vi "AlGaInPAs_v19e.vi"(2 "Debug Mode":bool, 3 "Elapsed Time(s)":dbl, 4 "State":enum16{"Edit", "Start", "Run", "End", "Idle"}(ring), 5 "Argument List In":string[](array[string])) -> (0 "Status Out":string, 1 "Argument List Out":string[](array[string]))   [LabVIEW 2011]
uses:
  high_level_proc/Al_bubbler.ctl
  high_level_proc/Ga_bubbler.ctl
  high_level_proc/In_bubbler.ctl
  high_level_proc/P_gas.ctl
  high_level_proc/As_gas.ctl
  high_level_proc/P_bubbler.ctl
panel:
  out "P bubbler Copy":T1 {"P bubbler main"."Flow" format="%.2f"}
  in  "P bubbler":T2 {"P bubbler main"."Flow" format="%.2f"}
  out "As gas Copy":T3 {"As gas main"."Flow" format="%.2f"}
  in  "As gas":T4 {"As gas main"."Flow" format="%.2f"}
  out "P gas Copy":T5 {"P gas main"."Flow" format="%.2f"}
  in  "P gas":T6 {"P gas main"."Flow" format="%.2f"}
  out "In bubbler Copy":T7 {"In main"."Flow" format="%.2f"}
  in  "In bubbler":T8 {"In main"."Flow" format="%.2f"}
  out "Ga bubbler Copy":T9={"Ga bubbler Active"=FALSE, "Ga main"={"Flow"=0.0, "Ga Run"=FALSE, "Prep Ga"=FALSE, "Dilution"=FALSE, "Ga Calculated"=1, "MFC2 flow"=10.0, "MFC3 flow"=100.0, "MFC1 flow"=0.0}} {"Ga main"."MFC1 flow" format="%.4f"; "Ga main"."MFC3 flow" format="%.1f"; "Ga main"."MFC2 flow" format="%.2f"; "Ga main"."Ga Calculated" items=["Ga flow", "MFC1", "MFC2", "MFC3"]; "Ga main"."Flow" format="%.2f"}
  in  "Ga bubbler":T10={"Ga bubbler Active"=FALSE, "Ga main"={"Flow"=0.0, "Ga Run"=FALSE, "Prep Ga"=FALSE, "Dilution"=FALSE, "Ga Calculated"=1, "MFC2 flow"=10.0, "MFC3 flow"=100.0, "MFC1 flow"=0.0}} {"Ga main"."MFC1 flow" format="%.4f"; "Ga main"."MFC3 flow" format="%.1f"; "Ga main"."MFC2 flow" format="%.2f"; "Ga main"."Ga Calculated" items=["Ga flow", "MFC1", "MFC2", "MFC3"]; "Ga main"."Flow" format="%.2f"}
  out "Al bubbler Copy":T11 {"Al main"."Al Flow" format="%.2f"}
  in  "Al bubbler":T12 {"Al main"."Al Flow" format="%.2f"}
  out "prep_done":bool
  out "run started":bool
  out "first":bool=TRUE
  out "total time":dbl
  out "is OK?":bool
  in  "prep_time":dbl
  in  "Cancel":bool
  in  "OK":bool
  out "tTotal(s) 2":dbl
  # "Add pre-run time to run time in editor."
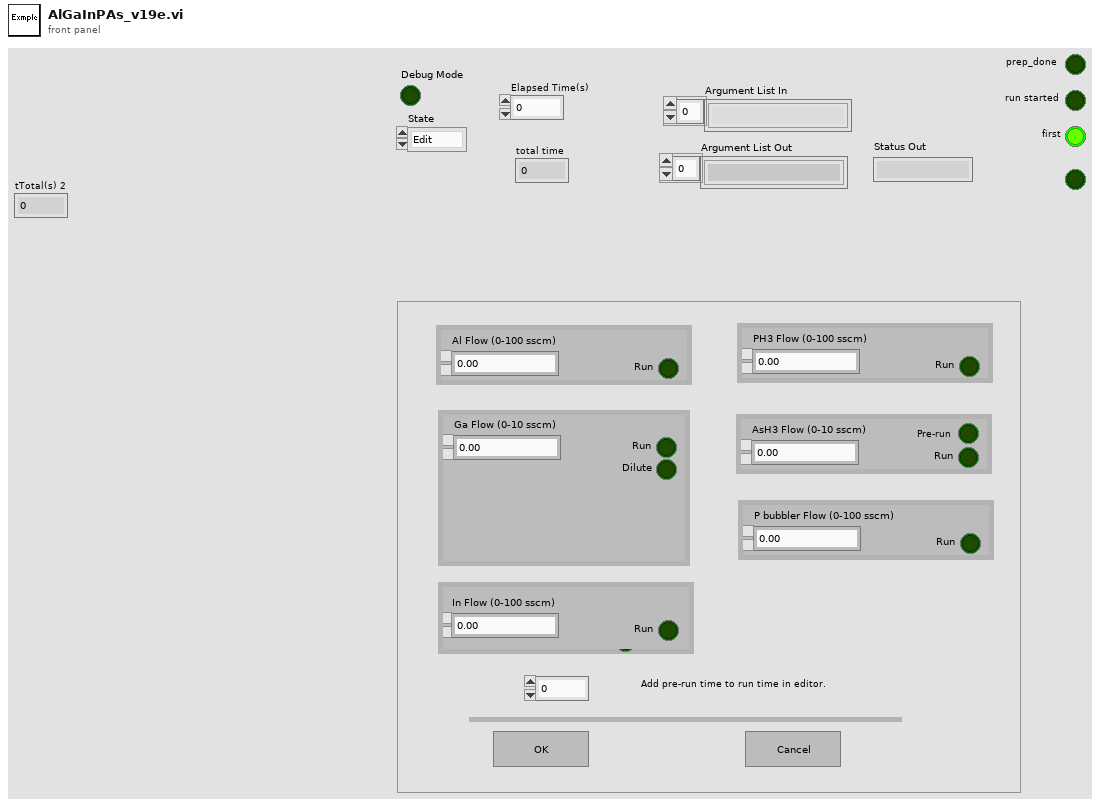
[diagram p1: front panel]
types:
  T1 = cluster{"P bubbler Active":bool, "P bubbler main":cluster{"Flow":dbl, "P bubbler Run":bool, "P bubbler Prep":bool}}
  T2 = typedef "P_bubbler.ctl" = cluster{"P bubbler Active":bool, "P bubbler main":cluster{"Flow":dbl, "P bubbler Run":bool, "P bubbler Prep":bool}}
  T3 = cluster{"As gas Active":bool, "As gas main":cluster{"Flow":dbl, "AsH3 Run":bool, "AsH3 Prep":bool}}
  T4 = typedef "As_gas.ctl" = cluster{"As gas Active":bool, "As gas main":cluster{"Flow":dbl, "AsH3 Run":bool, "AsH3 Prep":bool}}
  T5 = cluster{"P gas Active":bool, "P gas main":cluster{"Flow":dbl, "PH3 Run":bool, "PH3 Prep":bool}}
  T6 = typedef "P_gas.ctl" = cluster{"P gas Active":bool, "P gas main":cluster{"Flow":dbl, "PH3 Run":bool, "PH3 Prep":bool}}
  T7 = cluster{"In main":cluster{"Flow":dbl, "In Run":bool, "Prep In":bool}, "In bubbler Active":bool}
  T8 = typedef "In_bubbler.ctl" = cluster{"In main":cluster{"Flow":dbl, "In Run":bool, "Prep In":bool}, "In bubbler Active":bool}
  T9 = cluster{"Ga bubbler Active":bool, "Ga main":cluster{"Flow":dbl, "Ga Run":bool, "Prep Ga":bool, "Dilution":bool, "Ga Calculated":u16, "MFC2 flow":dbl, "MFC3 flow":dbl, "MFC1 flow":dbl}}
  T10 = typedef "Ga_bubbler.ctl" = cluster{"Ga bubbler Active":bool, "Ga main":cluster{"Flow":dbl, "Ga Run":bool, "Prep Ga":bool, "Dilution":bool, "Ga Calculated":u16, "MFC2 flow":dbl, "MFC3 flow":dbl, "MFC1 flow":dbl}}
  T11 = cluster{"Al Active":bool, "Al main":cluster{"Al Flow":dbl, "Al Run":bool, "Prep Al":bool}}
  T12 = typedef "Al_bubbler.ctl" = cluster{"Al Active":bool, "Al main":cluster{"Al Flow":dbl, "Al Run":bool, "Prep Al":bool}}
  T13 = enum16{"Discrete", "Continuous", "Instantaneous", "Finite"}
  T14 = enum32{"Invalid", "Default", "Floating", "Floating/Auto-Hide", "Modal"}
  T15 = enum8{"Enabled", "Disabled", "Disabled and Grayed Out"}
  T16 = cluster{"Al Flow":dbl, "Al Run":bool, "Prep Al":bool}
  T17 = cluster{"Flow":dbl, "Ga Run":bool, "Prep Ga":bool, "Dilution":bool, "Ga Calculated":u16, "MFC2 flow":dbl, "MFC3 flow":dbl, "MFC1 flow":dbl}
  T18 = cluster{"Flow":dbl, "In Run":bool, "Prep In":bool}
  T19 = cluster{"Flow":dbl, "PH3 Run":bool, "PH3 Prep":bool}
  T20 = cluster{"Flow":dbl, "AsH3 Run":bool, "AsH3 Prep":bool}
  T21 = cluster{"Flow":dbl, "P bubbler Run":bool, "P bubbler Prep":bool}
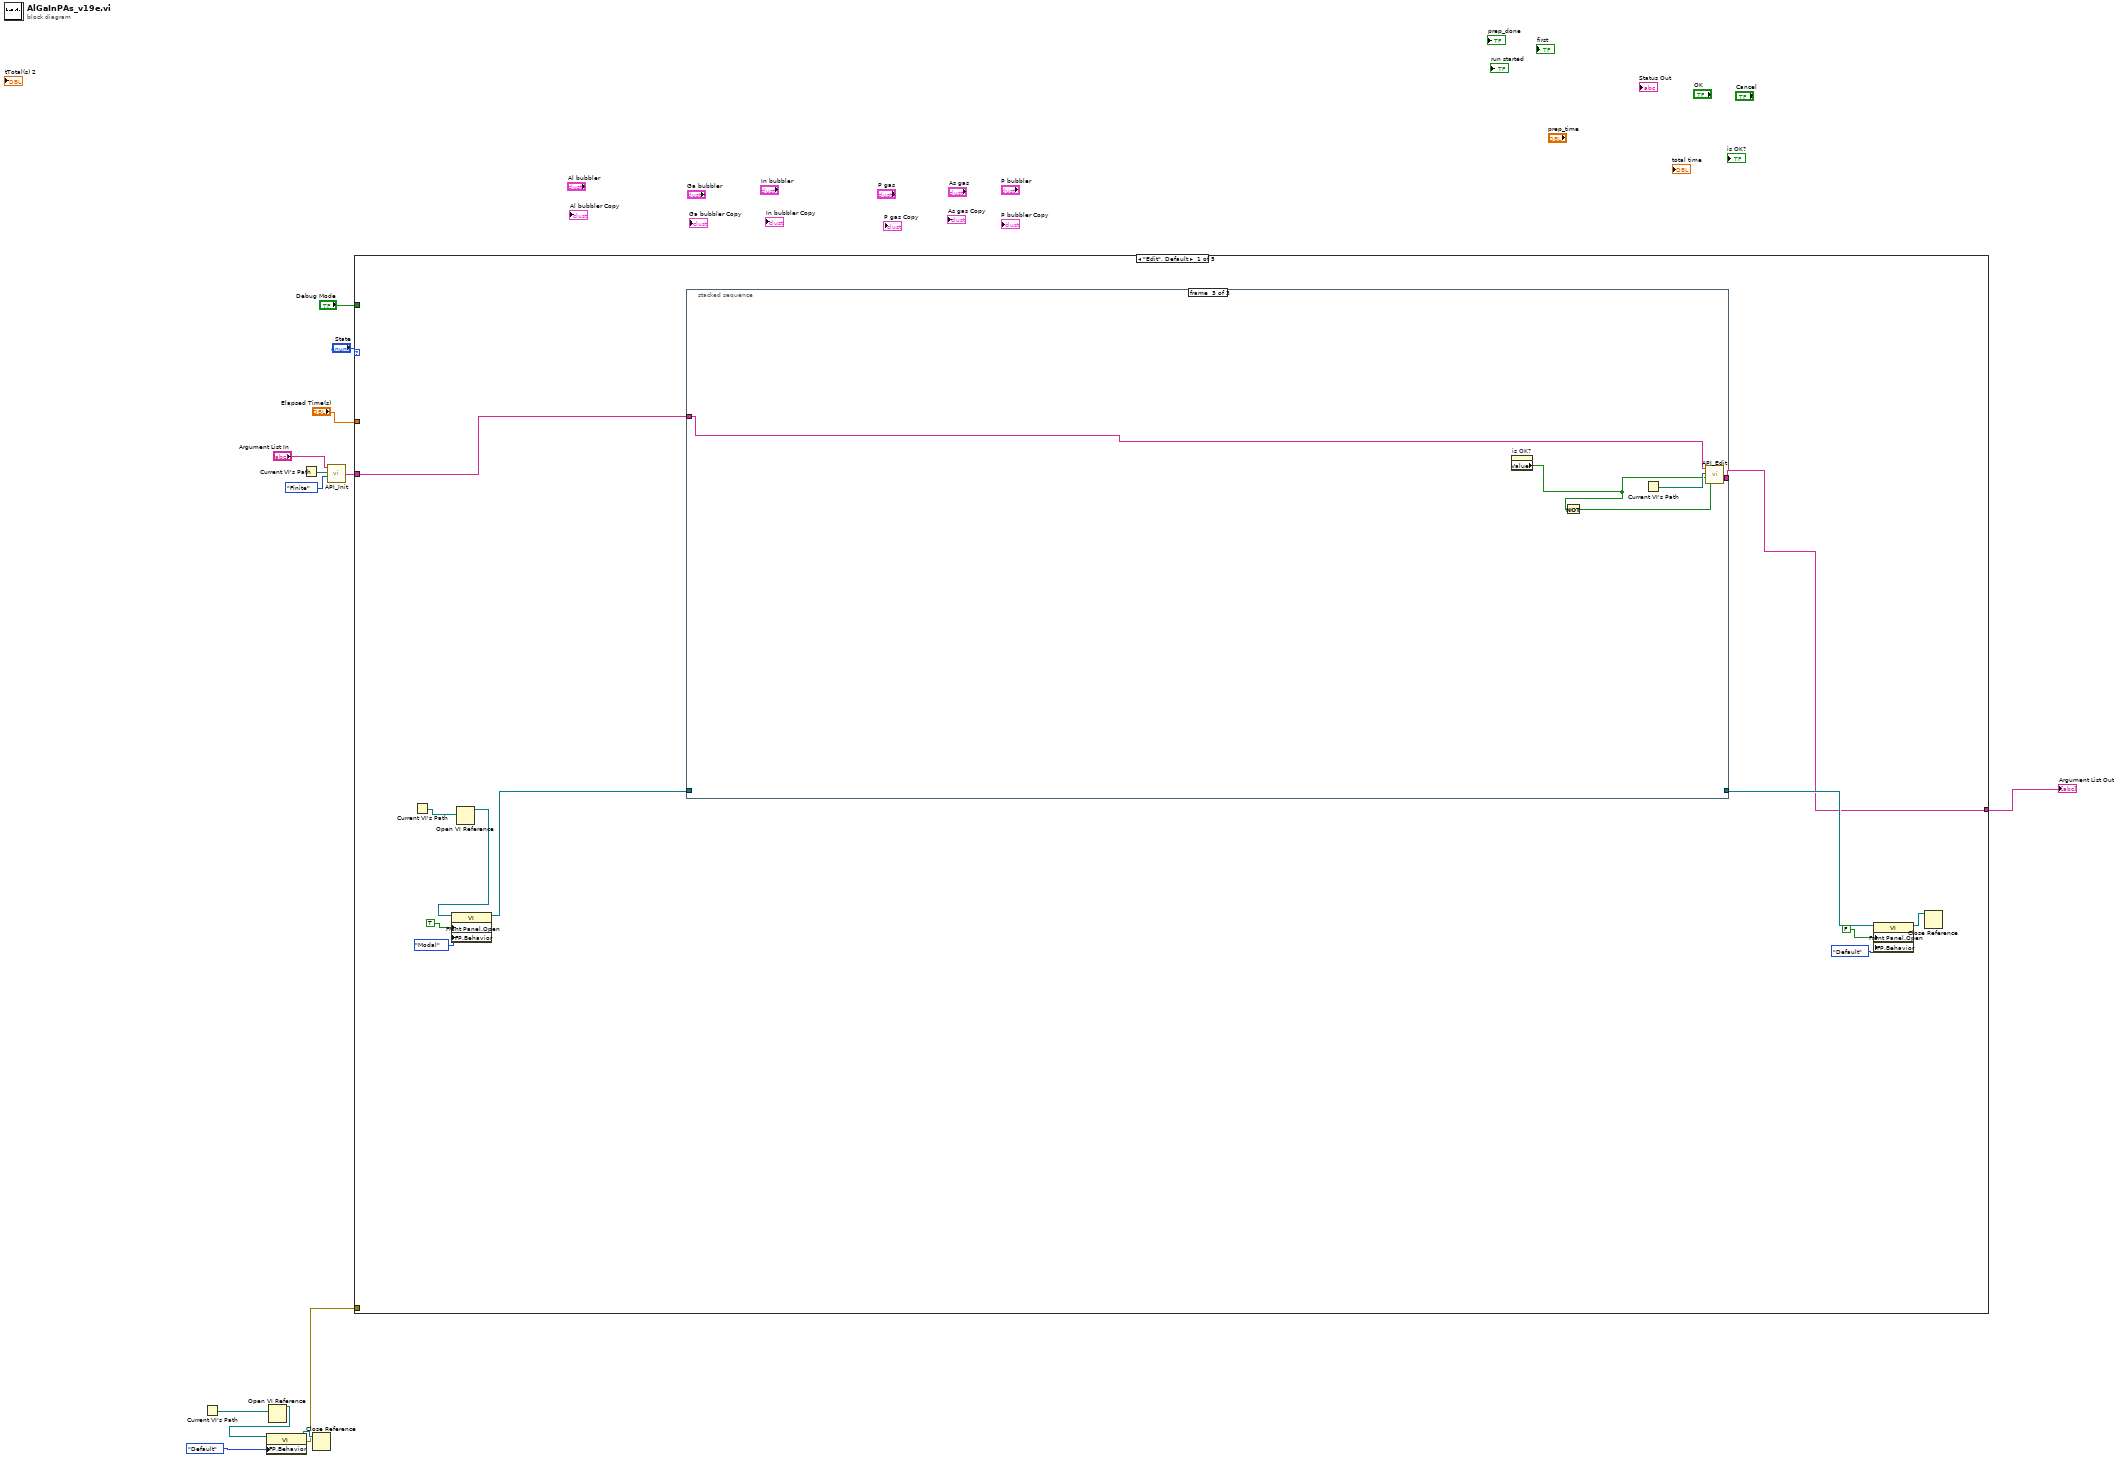
[diagram p0: block diagram]
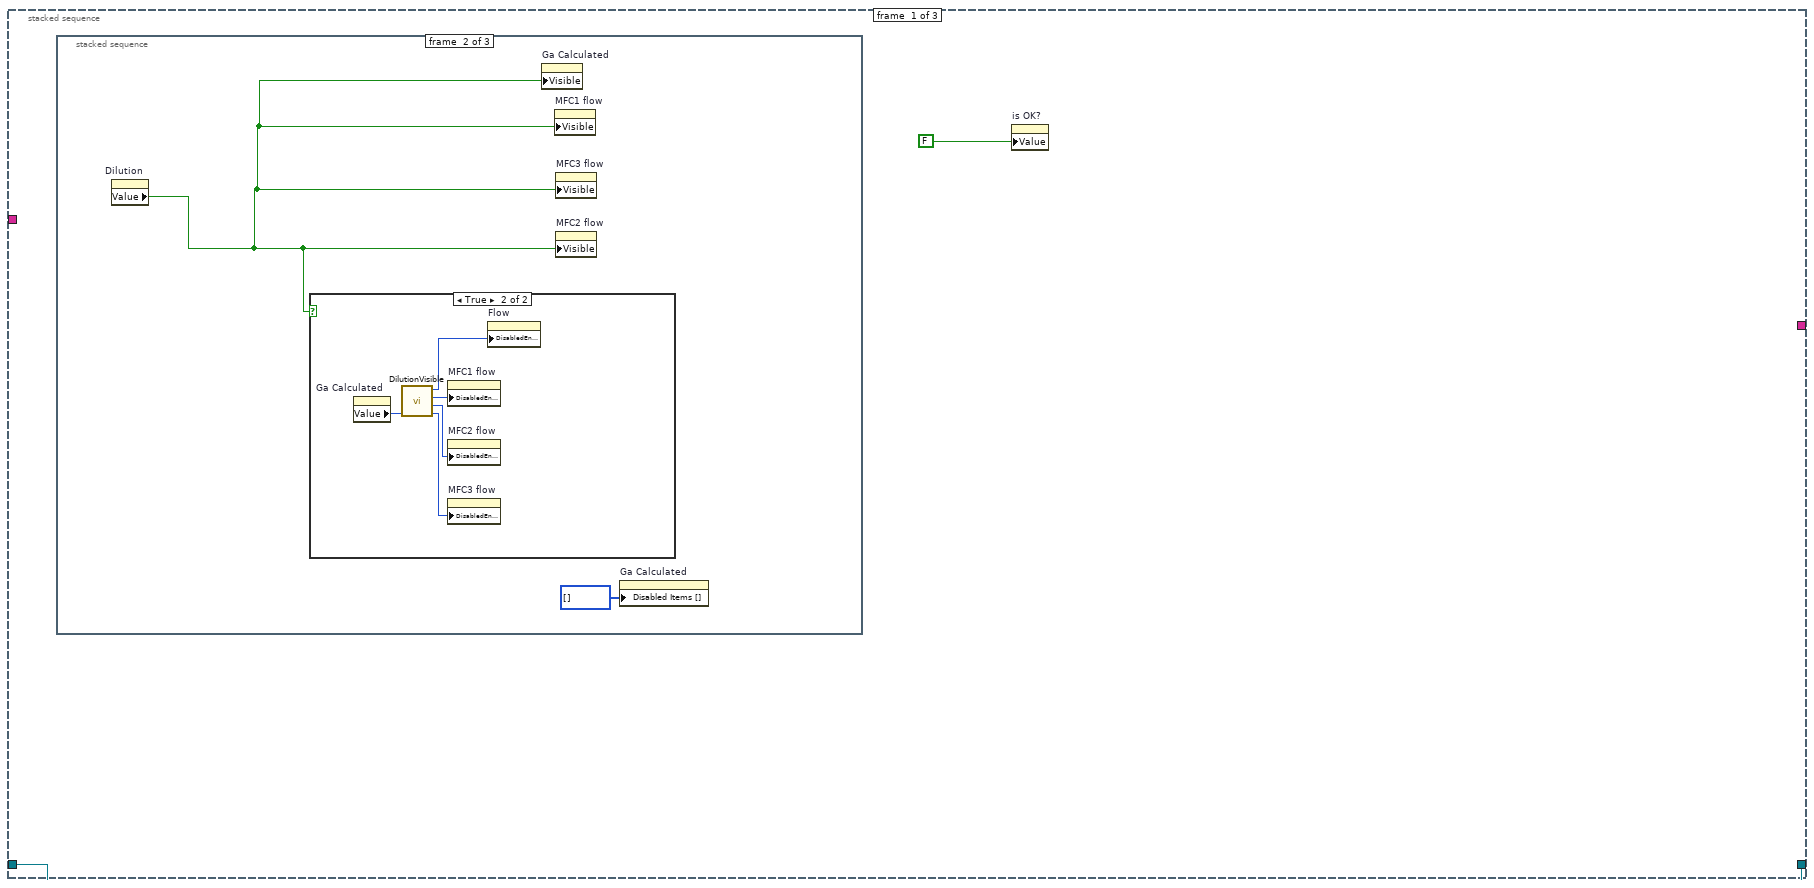
[diagram p2: hidden frame]
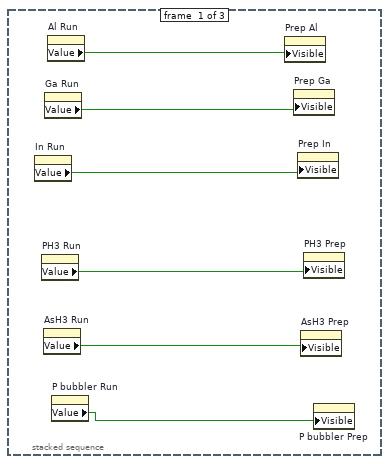
[diagram p3: hidden frame]
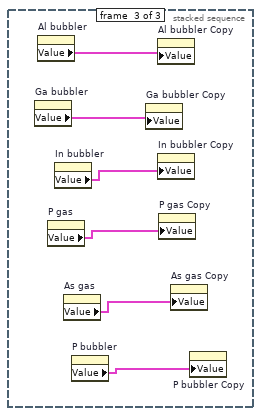
[diagram p5: hidden frame]
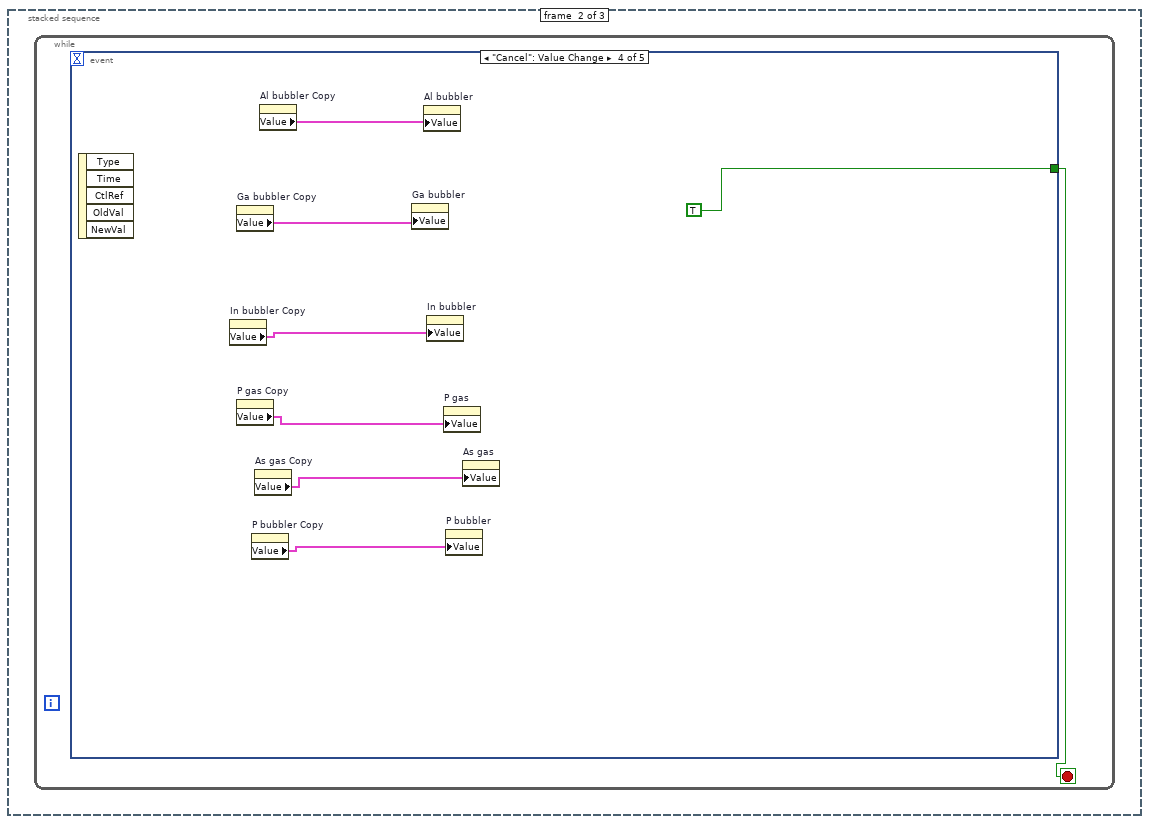
[diagram p6: hidden frame]
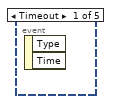
[diagram p7: hidden frame]
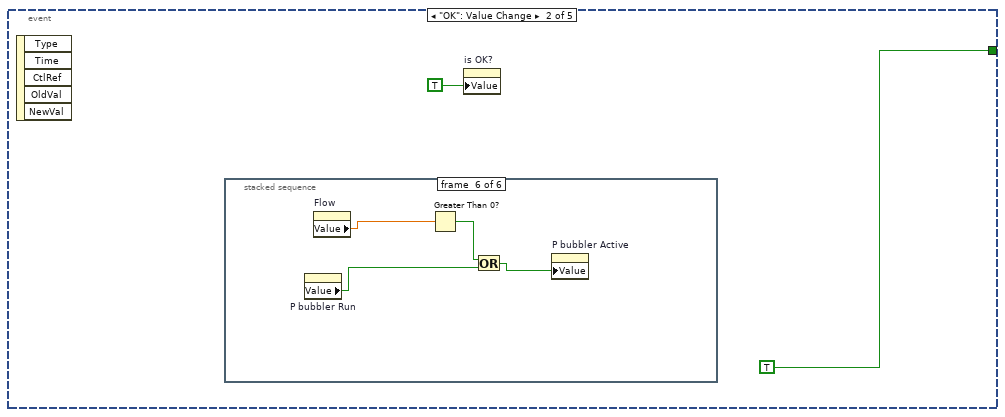
[diagram p8: hidden frame]
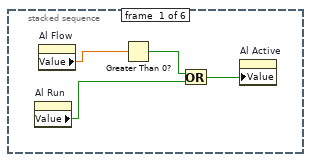
[diagram p9: hidden frame]
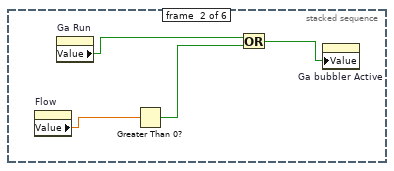
[diagram p10: hidden frame]
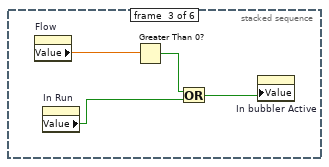
[diagram p11: hidden frame]
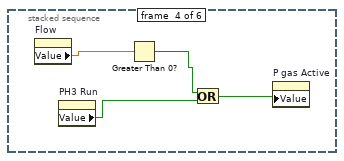
[diagram p12: hidden frame]
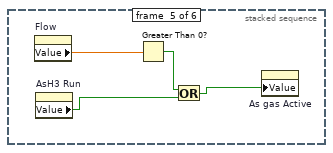
[diagram p13: hidden frame]
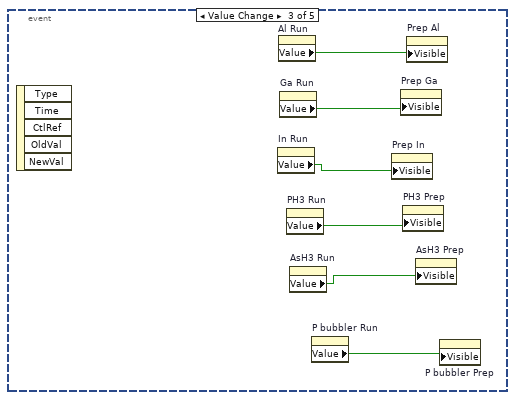
[diagram p14: hidden frame]
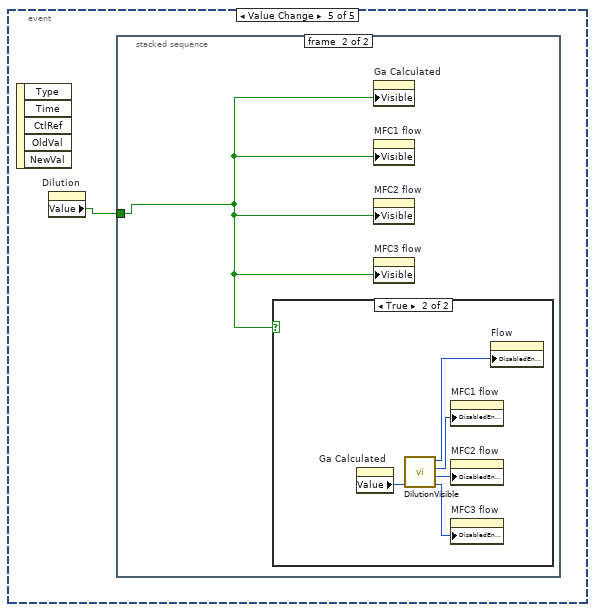
[diagram p15: hidden frame]
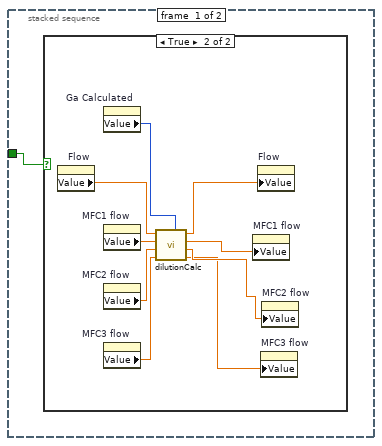
[diagram p16: hidden frame]
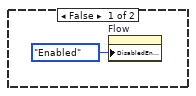
[diagram p18: hidden frame]
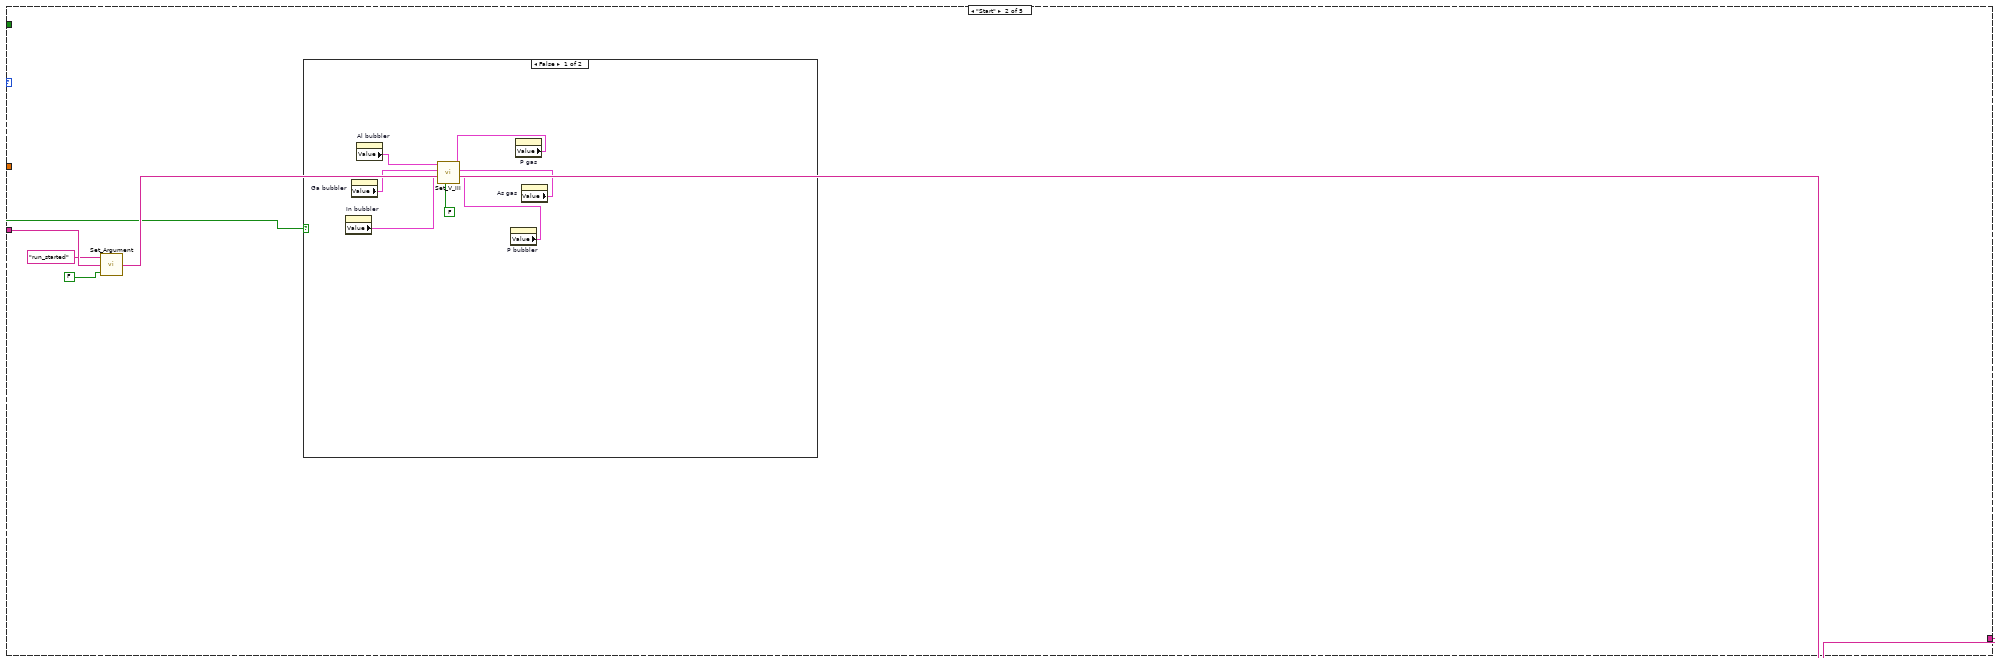
[diagram p19: hidden frame]
diagram:
  n1 = Current VI's Path() -> (path=w9:path)
  n2 = Open VI Reference(vi path=w9) -> (vi reference=w8:refnum<vi>)  [unwired: 1 in, 5 out]
  n3 = property class="VI"(reference=w8, "FP.Behavior"=T14."Default" ("Front Panel Window:Behavior")) -> (reference out=w6:refnum<vi>, error out=w5:errorcluster)  [unwired: 1 in]
  n4 = Current VI's Path() -> (path=w4:path)
  n5 = Close Reference(reference=w6) -> ()  [unwired: 1 in, 1 out]
  n6 = call "API_Init.vi"("API Mode"=T13."Finite", "VI Path"=w4, "Argument List In"="Argument List In") -> ("Argument List Out"=w1:string[])  [unwired: 1 in]
  n7 = case shown="\"Edit\", Default" "State" {
    tunnel: "Debug Mode" -> [_ w109 w123 _ _]
    tunnel: "Elapsed Time(s)" -> [_ _ w124 _ _]
    tunnel: w1 -> [w15 w111 w122 w222 w223]
    tunnel: [w14 w110 w121 w222 w223] -> w10
    tunnel: w5 -> [_ _ _ _ _]
    frame "Edit", Default {
      n8 = Current VI's Path() -> (path=w20:path)
      n9 = Open VI Reference(vi path=w20) -> (vi reference=w19:refnum<vi>)  [unwired: 1 in, 5 out]
      n10 = property class="VI"(reference=w19, "Front Panel.Open"=TRUE ("Front Panel Window:Open"), "FP.Behavior"=T14."Modal" ("Front Panel Window:Behavior")) -> (reference out=w18:refnum<vi>)  [unwired: 1 in, 1 out]
      n11 = stacked-sequence {
        tunnel: w15 -> [_ _ w105]
        tunnel: w18 -> [w26 _ _]
        tunnel: [w26 _ _] -> w22
        tunnel: [_ _ w106] -> w14
        frame #0 {
          n12 = stacked-sequence {
            frame #0 {
              n13 = property on="In Run" class="Bool (strict)"() -> ("Value"=w31:bool)  [unwired: 2 in, 2 out]
              n14 = property on="PH3 Run" class="Bool (strict)"() -> ("Value"=w29:bool)  [unwired: 2 in, 2 out]
              n15 = property on="AsH3 Run" class="Bool (strict)"() -> ("Value"=w28:bool)  [unwired: 2 in, 2 out]
              n16 = property on="Ga Run" class="Bool (strict)"() -> ("Value"=w30:bool)  [unwired: 2 in, 2 out]
              n17 = property on="Al Run" class="Bool (strict)"() -> ("Value"=w32:bool)  [unwired: 2 in, 2 out]
              n18 = property on="P bubbler Run" class="Bool (strict)"() -> ("Value"=w27:bool)  [unwired: 2 in, 2 out]
              n19 = property on="Prep Al" class="Bool (strict)"("Visible"=w32) -> ()  [unwired: 2 in, 2 out]
              n20 = property on="Prep Ga" class="Bool (strict)"("Visible"=w30) -> ()  [unwired: 2 in, 2 out]
              n21 = property on="Prep In" class="Bool (strict)"("Visible"=w31) -> ()  [unwired: 2 in, 2 out]
              n22 = property on="AsH3 Prep" class="Bool (strict)"("Visible"=w28) -> ()  [unwired: 2 in, 2 out]
              n23 = property on="PH3 Prep" class="Bool (strict)"("Visible"=w29) -> ()  [unwired: 2 in, 2 out]
              n24 = property on="P bubbler Prep" class="Bool (strict)"("Visible"=w27) -> ()  [unwired: 2 in, 2 out]
            }
            frame #1 {
              n25 = property on="Dilution" class="Bool (strict)"() -> ("Value"=w34:bool)  [unwired: 2 in, 2 out]
              n26 = case shown="True" w34 {
                frame False {
                }
                frame True {
                  n27 = property on="Ga Calculated" class="Ring (strict)"() -> ("Value"=w35:u16)  [unwired: 2 in, 2 out]
                  n28 = call "DilutionVisible.vi"("calculated"=w35) -> ("MFC3"=w38:u16, "MFC2"=w37:u16, "MFC1"=w36:u16, "flow"=w39:u16)  [unwired: 3 in]
                  n29 = property on="MFC1 flow" class="DigNum (strict)"("DisabledEnum"=w36) -> ()  [unwired: 2 in, 2 out]
                  n30 = property on="MFC2 flow" class="DigNum (strict)"("DisabledEnum"=w37) -> ()  [unwired: 2 in, 2 out]
                  n31 = property on="MFC3 flow" class="DigNum (strict)"("DisabledEnum"=w38) -> ()  [unwired: 2 in, 2 out]
                  n32 = property on="Flow" class="DigNum (strict)"("DisabledEnum"=w39) -> ()  [unwired: 2 in, 2 out]
                }
              }
              n33 = property on="Ga Calculated" class="Ring (strict)"("Visible"=w34) -> ()  [unwired: 2 in, 2 out]
              n34 = property on="MFC1 flow" class="DigNum (strict)"("Visible"=w34) -> ()  [unwired: 2 in, 2 out]
              n35 = property on="MFC3 flow" class="DigNum (strict)"("Visible"=w34) -> ()  [unwired: 2 in, 2 out]
              n36 = property on="MFC2 flow" class="DigNum (strict)"("Visible"=w34) -> ()  [unwired: 2 in, 2 out]
              n37 = property on="Ga Calculated" class="Ring (strict)"("Disabled Items []"=i32[] []) -> ()  [unwired: 2 in, 2 out]
            }
            frame #2 {
              n38 = property on="Ga bubbler" class="Clust (strict)"() -> ("Value"=w44:T9)  [unwired: 2 in, 2 out]
              n39 = property on="Al bubbler" class="Clust (strict)"() -> ("Value"=w45:T11)  [unwired: 2 in, 2 out]
              n40 = property on="P gas" class="Clust (strict)"() -> ("Value"=w42:T5)  [unwired: 2 in, 2 out]
              n41 = property on="In bubbler" class="Clust (strict)"() -> ("Value"=w43:T7)  [unwired: 2 in, 2 out]
              n42 = property on="As gas" class="Clust (strict)"() -> ("Value"=w41:T3)  [unwired: 2 in, 2 out]
              n43 = property on="P bubbler" class="Clust (strict)"() -> ("Value"=w40:T1)  [unwired: 2 in, 2 out]
              n44 = property on="Ga bubbler Copy" class="Clust (strict)"("Value"=w44) -> ()  [unwired: 2 in, 2 out]
              n45 = property on="Al bubbler Copy" class="Clust (strict)"("Value"=w45) -> ()  [unwired: 2 in, 2 out]
              n46 = property on="In bubbler Copy" class="Clust (strict)"("Value"=w43) -> ()  [unwired: 2 in, 2 out]
              n47 = property on="P gas Copy" class="Clust (strict)"("Value"=w42) -> ()  [unwired: 2 in, 2 out]
              n48 = property on="As gas Copy" class="Clust (strict)"("Value"=w41) -> ()  [unwired: 2 in, 2 out]
              n49 = property on="P bubbler Copy" class="Clust (strict)"("Value"=w40) -> ()  [unwired: 2 in, 2 out]
            }
          }
          n50 = property on="is OK?" class="Bool (strict)"("Value"=FALSE ("is OK?")) -> ()  [unwired: 2 in, 2 out]
        }
        frame #1 {
          n51 = while {
            stop <- w46 stop-if-true
            n52 = event shown="[3] \"Cancel\": Value Change" {
              selector: _ -> [_ _ _ _ _]
              dyn-events: _ -> [_ _ _ _ _]
              timeout: _ -> [_ _ _ _ _]
              tunnel: [_ TRUE _ TRUE _] -> w46
              event Timeout {
                n53 = event-data() -> ()  [unwired: 1 in, 2 out]
              }
              event "OK": Value Change {
                n54 = event-data() -> ()  [unwired: 1 in, 5 out]
                n55 = stacked-sequence {
                  frame #0 {
                    n56 = property on="Al Run" class="Bool (strict)"() -> ("Value"=w50:bool)  [unwired: 2 in, 2 out]
                    n57 = property on="Al Flow" class="DigNum (strict)"() -> ("Value"=w51:dbl)  [unwired: 2 in, 2 out]
                    n58 = Greater Than 0?(x=w51) -> (x > 0?=w52:bool)
                    n59 = Or(x=w52, y=w50) -> (x .or. y?=w49:bool)
                    n60 = property on="Al Active" class="Bool (strict)"("Value"=w49) -> ()  [unwired: 2 in, 2 out]
                  }
                  frame #1 {
                    n61 = property on="Flow" class="DigNum (strict)"() -> ("Value"=w53:dbl)  [unwired: 2 in, 2 out]
                    n62 = property on="Ga Run" class="Bool (strict)"() -> ("Value"=w54:bool)  [unwired: 2 in, 2 out]
                    n63 = Greater Than 0?(x=w53) -> (x > 0?=w56:bool)
                    n64 = Or(x=w54, y=w56) -> (x .or. y?=w55:bool)
                    n65 = property on="Ga bubbler Active" class="Bool (strict)"("Value"=w55) -> ()  [unwired: 2 in, 2 out]
                  }
                  frame #2 {
                    n66 = property on="Flow" class="DigNum (strict)"() -> ("Value"=w59:dbl)  [unwired: 2 in, 2 out]
                    n67 = property on="In Run" class="Bool (strict)"() -> ("Value"=w58:bool)  [unwired: 2 in, 2 out]
                    n68 = Greater Than 0?(x=w59) -> (x > 0?=w60:bool)
                    n69 = Or(x=w60, y=w58) -> (x .or. y?=w57:bool)
                    n70 = property on="In bubbler Active" class="Bool (strict)"("Value"=w57) -> ()  [unwired: 2 in, 2 out]
                  }
                  frame #3 {
                    n71 = property on="Flow" class="DigNum (strict)"() -> ("Value"=w63:dbl)  [unwired: 2 in, 2 out]
                    n72 = property on="PH3 Run" class="Bool (strict)"() -> ("Value"=w62:bool)  [unwired: 2 in, 2 out]
                    n73 = Greater Than 0?(x=w63) -> (x > 0?=w64:bool)
                    n74 = Or(x=w64, y=w62) -> (x .or. y?=w61:bool)
                    n75 = property on="P gas Active" class="Bool (strict)"("Value"=w61) -> ()  [unwired: 2 in, 2 out]
                  }
                  frame #4 {
                    n76 = property on="Flow" class="DigNum (strict)"() -> ("Value"=w67:dbl)  [unwired: 2 in, 2 out]
                    n77 = property on="AsH3 Run" class="Bool (strict)"() -> ("Value"=w66:bool)  [unwired: 2 in, 2 out]
                    n78 = Greater Than 0?(x=w67) -> (x > 0?=w68:bool)
                    n79 = Or(x=w68, y=w66) -> (x .or. y?=w65:bool)
                    n80 = property on="As gas Active" class="Bool (strict)"("Value"=w65) -> ()  [unwired: 2 in, 2 out]
                  }
                  frame #5 {
                    n81 = property on="P bubbler Run" class="Bool (strict)"() -> ("Value"=w70:bool)  [unwired: 2 in, 2 out]
                    n82 = property on="Flow" class="DigNum (strict)"() -> ("Value"=w71:dbl)  [unwired: 2 in, 2 out]
                    n83 = Greater Than 0?(x=w71) -> (x > 0?=w72:bool)
                    n84 = Or(x=w72, y=w70) -> (x .or. y?=w69:bool)
                    n85 = property on="P bubbler Active" class="Bool (strict)"("Value"=w69) -> ()  [unwired: 2 in, 2 out]
                  }
                }
                n86 = property on="is OK?" class="Bool (strict)"("Value"=TRUE ("is OK?")) -> ()  [unwired: 2 in, 2 out]
              }
              event Value Change {
                n87 = event-data() -> ()  [unwired: 1 in, 5 out]
                n88 = property on="In Run" class="Bool (strict)"() -> ("Value"=w75:bool)  [unwired: 2 in, 2 out]
                n89 = property on="Al Run" class="Bool (strict)"() -> ("Value"=w77:bool)  [unwired: 2 in, 2 out]
                n90 = property on="Ga Run" class="Bool (strict)"() -> ("Value"=w76:bool)  [unwired: 2 in, 2 out]
                n91 = property on="PH3 Run" class="Bool (strict)"() -> ("Value"=w74:bool)  [unwired: 2 in, 2 out]
                n92 = property on="AsH3 Run" class="Bool (strict)"() -> ("Value"=w73:bool)  [unwired: 2 in, 2 out]
                n93 = property on="P bubbler Run" class="Bool (strict)"() -> ("Value"=w78:bool)  [unwired: 2 in, 2 out]
                n94 = property on="Prep In" class="Bool (strict)"("Visible"=w75) -> ()  [unwired: 2 in, 2 out]
                n95 = property on="Prep Ga" class="Bool (strict)"("Visible"=w76) -> ()  [unwired: 2 in, 2 out]
                n96 = property on="PH3 Prep" class="Bool (strict)"("Visible"=w74) -> ()  [unwired: 2 in, 2 out]
                n97 = property on="Prep Al" class="Bool (strict)"("Visible"=w77) -> ()  [unwired: 2 in, 2 out]
                n98 = property on="AsH3 Prep" class="Bool (strict)"("Visible"=w73) -> ()  [unwired: 2 in, 2 out]
                n99 = property on="P bubbler Prep" class="Bool (strict)"("Visible"=w78) -> ()  [unwired: 2 in, 2 out]
              }
              event "Cancel": Value Change {
                n100 = event-data() -> ()  [unwired: 1 in, 5 out]
                n101 = property on="In bubbler Copy" class="Clust (strict)"() -> ("Value"=w83:T7)  [unwired: 2 in, 2 out]
                n102 = property on="Ga bubbler Copy" class="Clust (strict)"() -> ("Value"=w82:T9)  [unwired: 2 in, 2 out]
                n103 = property on="P gas Copy" class="Clust (strict)"() -> ("Value"=w81:T5)  [unwired: 2 in, 2 out]
                n104 = property on="P bubbler Copy" class="Clust (strict)"() -> ("Value"=w79:T1)  [unwired: 2 in, 2 out]
                n105 = property on="As gas Copy" class="Clust (strict)"() -> ("Value"=w80:T3)  [unwired: 2 in, 2 out]
                n106 = property on="Al bubbler Copy" class="Clust (strict)"() -> ("Value"=w84:T11)  [unwired: 2 in, 2 out]
                n107 = property on="Ga bubbler" class="Clust (strict)"("Value"=w82) -> ()  [unwired: 2 in, 2 out]
                n108 = property on="Al bubbler" class="Clust (strict)"("Value"=w84) -> ()  [unwired: 2 in, 2 out]
                n109 = property on="In bubbler" class="Clust (strict)"("Value"=w83) -> ()  [unwired: 2 in, 2 out]
                n110 = property on="P gas" class="Clust (strict)"("Value"=w81) -> ()  [unwired: 2 in, 2 out]
                n111 = property on="P bubbler" class="Clust (strict)"("Value"=w79) -> ()  [unwired: 2 in, 2 out]
                n112 = property on="As gas" class="Clust (strict)"("Value"=w80) -> ()  [unwired: 2 in, 2 out]
              }
              event Value Change {
                n113 = event-data() -> ()  [unwired: 1 in, 5 out]
                n114 = property on="Dilution" class="Bool (strict)"() -> ("Value"=w86:bool)  [unwired: 2 in, 2 out]
                n115 = stacked-sequence {
                  tunnel: w86 -> [w87 w97]
                  frame #0 {
                    n116 = case shown="True" w87 {
                      frame False {
                      }
                      frame True {
                        n117 = property on="Flow" class="DigNum (strict)"() -> ("Value"=w95:dbl)  [unwired: 2 in, 2 out]
                        n118 = property on="Ga Calculated" class="Ring (strict)"() -> ("Value"=w96:u16)  [unwired: 2 in, 2 out]
                        n119 = property on="MFC1 flow" class="DigNum (strict)"() -> ("Value"=w94:dbl)  [unwired: 2 in, 2 out]
                        n120 = property on="MFC2 flow" class="DigNum (strict)"() -> ("Value"=w93:dbl)  [unwired: 2 in, 2 out]
                        n121 = property on="MFC3 flow" class="DigNum (strict)"() -> ("Value"=w92:dbl)  [unwired: 2 in, 2 out]
                        n122 = call "dilutionCalc.vi"("Calculated"=w96, "MFC3"=w92, "MFC2"=w93, "MFC1"=w94, "flow"=w95) -> ("MFC3 out"=w88:dbl, "MFC2 out"=w89:dbl, "MFC1 out"=w90:dbl, "flow out"=w91:dbl)  [unwired: 1 in]
                        n123 = property on="MFC1 flow" class="DigNum (strict)"("Value"=w90) -> ()  [unwired: 2 in, 2 out]
                        n124 = property on="Flow" class="DigNum (strict)"("Value"=w91) -> ()  [unwired: 2 in, 2 out]
                        n125 = property on="MFC3 flow" class="DigNum (strict)"("Value"=w88) -> ()  [unwired: 2 in, 2 out]
                        n126 = property on="MFC2 flow" class="DigNum (strict)"("Value"=w89) -> ()  [unwired: 2 in, 2 out]
                      }
                    }
                  }
                  frame #1 {
                    n127 = case shown="True" w97 {
                      frame False {
                        n128 = property on="Flow" class="DigNum (strict)"("DisabledEnum"=T15."Enabled" ("Disabled")) -> ()  [unwired: 2 in, 2 out]
                      }
                      frame True {
                        n129 = property on="Ga Calculated" class="Ring (strict)"() -> ("Value"=w99:u16)  [unwired: 2 in, 2 out]
                        n130 = call "DilutionVisible.vi"("calculated"=w99) -> ("MFC3"=w103:u16, "MFC2"=w102:u16, "MFC1"=w101:u16, "flow"=w100:u16)  [unwired: 3 in]
                        n131 = property on="MFC1 flow" class="DigNum (strict)"("DisabledEnum"=w101) -> ()  [unwired: 2 in, 2 out]
                        n132 = property on="MFC2 flow" class="DigNum (strict)"("DisabledEnum"=w102) -> ()  [unwired: 2 in, 2 out]
                        n133 = property on="MFC3 flow" class="DigNum (strict)"("DisabledEnum"=w103) -> ()  [unwired: 2 in, 2 out]
                        n134 = property on="Flow" class="DigNum (strict)"("DisabledEnum"=w100) -> ()  [unwired: 2 in, 2 out]
                      }
                    }
                    n135 = property on="Ga Calculated" class="Ring (strict)"("Visible"=w97) -> ()  [unwired: 2 in, 2 out]
                    n136 = property on="MFC1 flow" class="DigNum (strict)"("Visible"=w97) -> ()  [unwired: 2 in, 2 out]
                    n137 = property on="MFC2 flow" class="DigNum (strict)"("Visible"=w97) -> ()  [unwired: 2 in, 2 out]
                    n138 = property on="MFC3 flow" class="DigNum (strict)"("Visible"=w97) -> ()  [unwired: 2 in, 2 out]
                  }
                }
              }
            }
          }
        }
        frame #2 {
          n139 = property on="is OK?" class="Bool (strict)"() -> ("Value"=w104:bool)  [unwired: 2 in, 2 out]
          n140 = Not(x=w104) -> (.not. x?=w108:bool)
          n141 = Current VI's Path() -> (path=w107:path)
          n142 = call "API_Edit.vi"("Cancel"=w108, "OK"=w104, "VI Path"=w107, "Argument List In"=w105) -> ("Argument List Out"=w106:string[])
        }
      }
      n143 = property class="VI"(reference=w22, "Front Panel.Open"=FALSE ("Front Panel Window:Open"), "FP.Behavior"=T14."Default" ("Front Panel Window:Behavior")) -> (reference out=w23:refnum<vi>)  [unwired: 1 in, 1 out]
      n144 = Close Reference(reference=w23) -> ()  [unwired: 1 in, 1 out]
    }
    frame "Start" {
      n145 = call "Set_Argument.vi"("Enable"=FALSE, "Argument"="run_started", "Argument List In"=w111) -> ("Argument List Out"=w110:string[])
      n146 = case shown="False" w109 {
        frame False {
          n147 = property on="In bubbler" class="Clust (strict)"() -> ("Value"=w118:T7)  [unwired: 2 in, 2 out]
          n148 = property on="Ga bubbler" class="Clust (strict)"() -> ("Value"=w119:T9)  [unwired: 2 in, 2 out]
          n149 = property on="Al bubbler" class="Clust (strict)"() -> ("Value"=w120:T11)  [unwired: 2 in, 2 out]
          n150 = property on="P bubbler" class="Clust (strict)"() -> ("Value"=w115:T1)  [unwired: 2 in, 2 out]
          n151 = property on="P gas" class="Clust (strict)"() -> ("Value"=w117:T5)  [unwired: 2 in, 2 out]
          n152 = property on="As gas" class="Clust (strict)"() -> ("Value"=w116:T3)  [unwired: 2 in, 2 out]
          n153 = call "Set_V_III.vi"("P bubbler"=w115, "As gas"=w116, "P gas"=w117, "Run Started"=FALSE, "In bubbler"=w118, "Ga bubbler"=w119, "Al bubbler"=w120) -> ()  [unwired: 5 in]
        }
        frame True {
        }
      }
    }
    frame "Run" {
      n154 = stacked-sequence {
        tunnel: w124 -> [_ w129 _ _]
        tunnel: w122 -> [w126 _ _ w200]
        tunnel: w123 -> [_ _ _ w198]
        tunnel: [_ _ _ w199] -> w121
        frame #0 {
          n155 = call "Get_Argument.vi"("Argument"="run_started", "Argument List"=w126) -> ("Enabled"=w125:bool)
          n156 = local write "run started"(w125) -> ()
        }
        frame #1 {
          n157 = property on="prep_time" class="DigNum (strict)"() -> ("Value"=w130:dbl)  [unwired: 2 in, 2 out]
          n158 = Greater Or Equal?(x=w129, y=w130) -> (x >= y?=w128:bool)
          n159 = local write "prep_done"(w128) -> ()
        }
        frame #2 {
          n160 = local read "run started"() -> (w132:bool)
          n161 = Not(x=w132) -> (.not. x?=w131:bool)
          n162 = stacked-sequence {
            tunnel: w131 -> [w134 w141 w151 w161 w171 w181 w191]
            frame #0 {
              n163 = case shown="False" w134 {
                tunnel: ["run: " "pre-run: "] -> w133
                frame False {
                }
                frame True {
                }
              }
              n164 = property on="Status Out" class="Str"("Value"=w133) -> ()  [unwired: 2 in, 2 out]
            }
            frame #1 {
              n165 = property on="Al main" class="Clust (strict)"() -> ("Value"=w139:T16)  [unwired: 2 in, 2 out]
              n166 = property on="Al Active" class="Bool (strict)"() -> ("Value"=w140:bool)  [unwired: 2 in, 2 out]
              n167 = property on="Status Out" class="Str"() -> ("Value"=w146:string)  [unwired: 2 in, 2 out]
              n168 = Unbundle By Name(w139) -> ("Al Run"=w138:bool, "Prep Al"=w137:bool)
              n169 = call "flow_strings.vi"("string in"=w146, "is first in?"=TRUE, "use source?"=w140, "name"="Al", "run source?"=w138, "prep source?"=w137, "is prep?"=w141) -> ("string out"=w145:string, "is first out?"=w144:bool)
              n170 = property on="Status Out" class="Str"("Value"=w145) -> ()  [unwired: 2 in, 2 out]
              n171 = property on="first" class="Bool (strict)"("Value"=w144) -> ()  [unwired: 2 in, 2 out]
            }
            frame #2 {
              n172 = property on="Ga main" class="Clust (strict)"() -> ("Value"=w149:T17)  [unwired: 2 in, 2 out]
              n173 = property on="Ga bubbler Active" class="Bool (strict)"() -> ("Value"=w150:bool)  [unwired: 2 in, 2 out]
              n174 = property on="first" class="Bool (strict)"() -> ("Value"=w153:bool)  [unwired: 2 in, 2 out]
              n175 = property on="Status Out" class="Str"() -> ("Value"=w155:string)  [unwired: 2 in, 2 out]
              n176 = Unbundle By Name(w149) -> ("Ga Run"=w148:bool, "Prep Ga"=w147:bool)
              n177 = call "flow_strings.vi"("string in"=w155, "is first in?"=w153, "use source?"=w150, "name"="Ga", "run source?"=w148, "prep source?"=w147, "is prep?"=w151) -> ("string out"=w156:string, "is first out?"=w152:bool)
              n178 = property on="Status Out" class="Str"("Value"=w156) -> ()  [unwired: 2 in, 2 out]
              n179 = property on="first" class="Bool (strict)"("Value"=w152) -> ()  [unwired: 2 in, 2 out]
            }
            frame #3 {
              n180 = property on="In bubbler Active" class="Bool (strict)"() -> ("Value"=w160:bool)  [unwired: 2 in, 2 out]
              n181 = property on="In main" class="Clust (strict)"() -> ("Value"=w159:T18)  [unwired: 2 in, 2 out]
              n182 = property on="first" class="Bool (strict)"() -> ("Value"=w164:bool)  [unwired: 2 in, 2 out]
              n183 = property on="Status Out" class="Str"() -> ("Value"=w166:string)  [unwired: 2 in, 2 out]
              n184 = Unbundle By Name(w159) -> ("In Run"=w158:bool, "Prep In"=w157:bool)
              n185 = call "flow_strings.vi"("string in"=w166, "is first in?"=w164, "use source?"=w160, "name"="In", "run source?"=w158, "prep source?"=w157, "is prep?"=w161) -> ("string out"=w163:string, "is first out?"=w162:bool)
              n186 = property on="Status Out" class="Str"("Value"=w163) -> ()  [unwired: 2 in, 2 out]
              n187 = property on="first" class="Bool (strict)"("Value"=w162) -> ()  [unwired: 2 in, 2 out]
            }
            frame #4 {
              n188 = property on="P gas Active" class="Bool (strict)"() -> ("Value"=w170:bool)  [unwired: 2 in, 2 out]
              n189 = property on="P gas main" class="Clust (strict)"() -> ("Value"=w169:T19)  [unwired: 2 in, 2 out]
              n190 = property on="first" class="Bool (strict)"() -> ("Value"=w173:bool)  [unwired: 2 in, 2 out]
              n191 = property on="Status Out" class="Str"() -> ("Value"=w175:string)  [unwired: 2 in, 2 out]
              n192 = Unbundle By Name(w169) -> ("PH3 Run"=w168:bool, "PH3 Prep"=w167:bool)
              n193 = call "flow_strings.vi"("string in"=w175, "is first in?"=w173, "use source?"=w170, "name"="PH3", "run source?"=w168, "prep source?"=w167, "is prep?"=w171) -> ("string out"=w174:string, "is first out?"=w172:bool)
              n194 = property on="Status Out" class="Str"("Value"=w174) -> ()  [unwired: 2 in, 2 out]
              n195 = property on="first" class="Bool (strict)"("Value"=w172) -> ()  [unwired: 2 in, 2 out]
            }
            frame #5 {
              n196 = property on="As gas Active" class="Bool (strict)"() -> ("Value"=w180:bool)  [unwired: 2 in, 2 out]
              n197 = property on="As gas main" class="Clust (strict)"() -> ("Value"=w179:T20)  [unwired: 2 in, 2 out]
              n198 = property on="first" class="Bool (strict)"() -> ("Value"=w183:bool)  [unwired: 2 in, 2 out]
              n199 = property on="Status Out" class="Str"() -> ("Value"=w185:string)  [unwired: 2 in, 2 out]
              n200 = Unbundle By Name(w179) -> ("AsH3 Run"=w178:bool, "AsH3 Prep"=w177:bool)
              n201 = call "flow_strings.vi"("string in"=w185, "is first in?"=w183, "use source?"=w180, "name"="AsH3", "run source?"=w178, "prep source?"=w177, "is prep?"=w181) -> ("string out"=w182:string, "is first out?"=w184:bool)
              n202 = property on="Status Out" class="Str"("Value"=w182) -> ()  [unwired: 2 in, 2 out]
              n203 = property on="first" class="Bool (strict)"("Value"=w184) -> ()  [unwired: 2 in, 2 out]
            }
            frame #6 {
              n204 = property on="P bubbler main" class="Clust (strict)"() -> ("Value"=w189:T21)  [unwired: 2 in, 2 out]
              n205 = property on="P bubbler Active" class="Bool (strict)"() -> ("Value"=w190:bool)  [unwired: 2 in, 2 out]
              n206 = Unbundle By Name(w189) -> ("P bubbler Run"=w188:bool, "P bubbler Prep"=w187:bool)
              n207 = property on="first" class="Bool (strict)"() -> ("Value"=w194:bool)  [unwired: 2 in, 2 out]
              n208 = property on="Status Out" class="Str"() -> ("Value"=w196:string)  [unwired: 2 in, 2 out]
              n209 = call "flow_strings.vi"("string in"=w196, "is first in?"=w194, "use source?"=w190, "name"="P liq", "run source?"=w188, "prep source?"=w187, "is prep?"=w191) -> ("string out"=w193:string, "is first out?"=w192:bool)
              n210 = property on="Status Out" class="Str"("Value"=w193) -> ()  [unwired: 2 in, 2 out]
              n211 = property on="first" class="Bool (strict)"("Value"=w192) -> ()  [unwired: 2 in, 2 out]
            }
          }
        }
        frame #3 {
          n212 = property on="prep_done" class="Bool (strict)"() -> ("Value"=w203:bool)  [unwired: 2 in, 2 out]
          n213 = property on="run started" class="Bool (strict)"() -> ("Value"=w202:bool)  [unwired: 2 in, 2 out]
          n214 = Not(x=w202) -> (.not. x?=w201:bool)
          n215 = And(x=w203, y=w201) -> (x .and. y?=w197:bool)
          n216 = case shown="True" w197 {
            selector: w197 -> [_ w205]
            tunnel: w200 -> [w204 w208]
            tunnel: [w204 w207] -> w199
            tunnel: w198 -> [_ w206]
            frame False {
            }
            frame True {
              n217 = stacked-sequence {
                tunnel: w206 -> [w210 _]
                tunnel: w208 -> [_ w219]
                tunnel: [_ w218] -> w207
                tunnel: w205 -> [w209 _]
                frame #0 {
                  n218 = case shown="False" w210 {
                    tunnel: w209 -> [w211 _]
                    frame False {
                      n219 = property on="In bubbler" class="Clust (strict)"() -> ("Value"=w215:T7)  [unwired: 2 in, 2 out]
                      n220 = property on="Ga bubbler" class="Clust (strict)"() -> ("Value"=w216:T9)  [unwired: 2 in, 2 out]
                      n221 = property on="Al bubbler" class="Clust (strict)"() -> ("Value"=w217:T11)  [unwired: 2 in, 2 out]
                      n222 = property on="P gas" class="Clust (strict)"() -> ("Value"=w214:T5)  [unwired: 2 in, 2 out]
                      n223 = property on="As gas" class="Clust (strict)"() -> ("Value"=w213:T3)  [unwired: 2 in, 2 out]
                      n224 = property on="P bubbler" class="Clust (strict)"() -> ("Value"=w212:T1)  [unwired: 2 in, 2 out]
                      n225 = call "Set_V_III.vi"("P bubbler"=w212, "As gas"=w213, "P gas"=w214, "Run Started"=w211, "In bubbler"=w215, "Ga bubbler"=w216, "Al bubbler"=w217) -> ()  [unwired: 5 in]
                    }
                    frame True {
                    }
                  }
                }
                frame #1 {
                  n226 = call "Set_Argument.vi"("Enable"=TRUE, "Argument"="run_started", "Argument List In"=w219) -> ("Argument List Out"=w218:string[])
                }
              }
            }
          }
        }
      }
    }
    frame "End" {
    }
    frame "Idle" {
    }
  }
  "Argument List Out" <- w10
